vi "Begin.vi"(8 "error in":errorcluster) -> (0 "error out":errorcluster)   [LabVIEW 2015]
doc: "Called before other user functions, this VI is expected to open initial I/O refnums, load in file data, and do all program initialization. Notice that the <B>error out</B> terminal is simply used for data flow. Wiring it to other structures or subVIs ensures that this VI runs first."
uses:
  <vilib>/Rock Robotics/WPI/DriverStation/WPI_DriverStationRobotMode2.ctl
  <vilib>/Rock Robotics/WPI/Joystick/WPI_JoystickDeviceEnum.ctl
  <vilib>/Rock Robotics/WPI/CAN/TalonSRX/WPI_CANTalonSRX_APIControlMode.ctl
  <vilib>/Rock Robotics/WPI/CAN/TalonSRX/WPI_CANTalonSRX_APIFeedbackSelect.ctl
  <vilib>/Rock Robotics/SystemInterfaces/DIO/FPGA_DIOPWMChannel.ctl
  <vilib>/Rock Robotics/WPI/SafetyOutput/WPI_SafetyOutputConfigMenu.ctl
  <vilib>/Rock Robotics/SystemInterfaces/spilib/spi_bus.ctl
  Robot Global Data.vi
  <vilib>/Rock Robotics/WPI/MotorControl/WPI_MotorControlOpenCANTalonSRX.vi
  <vilib>/Rock Robotics/WPI/MotorControl/WPI_MotorControlOpen VictorSP.vi
  <vilib>/Rock Robotics/WPI/Solenoid/WPI_SolenoidOpenSingle.vi
  <vilib>/Rock Robotics/WPI/RobotDrive/WPI_RobotDriveOpen2MotorWithVictorSP.vi
  Z navX/navX Library v2/IO/Open/Z900_navX_Open_SPI.vi
  <vilib>/Rock Robotics/Network Tables/NT Write String Array.vi
  <vilib>/Rock Robotics/WPI/Counter/WPI_CounterDigitalInputToDigitalSource.vi
  <vilib>/Rock Robotics/SystemInterfaces/DIO/FPGA_DIOChannel.ctl
  <vilib>/Rock Robotics/WPI/Encoder/WPI_EncoderType.ctl
  Z navX/navX Library v2/navX Library v2.lvlib
panel:
  in  "I 4":dbl
  in  "F 4":dbl=0.01
  in  "D 4":dbl caption="D"
  in  "P 4":dbl=1.0 caption="P"
  in  "Reverse Feedback Sensor 4":bool
  in  "I 3":dbl
  in  "F 3":dbl=0.01
  in  "D 3":dbl caption="D"
  in  "P 3":dbl=1.0 caption="P"
  in  "Reverse Feedback Sensor 3":bool
  in  "Encoder Codes Per Rev 3":u16=360
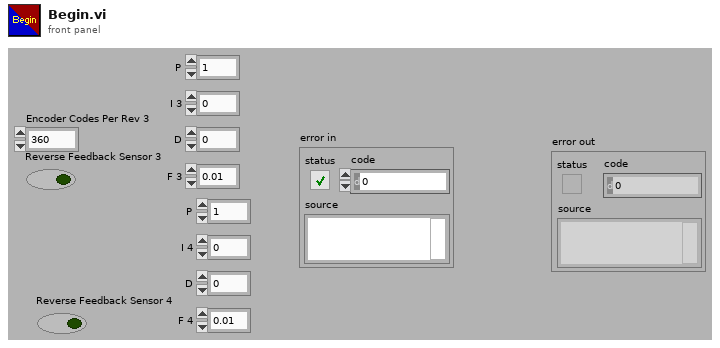
[diagram p1: front panel]
types:
  T1 = typedef "spi_bus.ctl" = enum16{"SPI On-Board, CS0", "SPI On-Board, CS1", "SPI On-Board, CS2", "SPI On-Board, CS3", "SPI MXP", "Invalid"}
  T2 = typedef "WPI_SafetyOutputConfigMenu.ctl" = enum16{"Enable", "Disable"}
  T3 = typedef "FPGA_DIOPWMChannel.ctl" = enum8{"PWM 0", "PWM 1", "PWM 2", "PWM 3", "PWM 4", "PWM 5", "PWM 6", "PWM 7", "PWM 8", "PWM 9", "PWM MXP 0", "PWM MXP 1", "PWM MXP 2", "PWM MXP 3", "PWM MXP 4", "PWM MXP 5", "PWM MXP 6", "PWM MXP 7", "PWM MXP 8", "PWM MXP 9", "Invalid"}
  T4 = typedef "WPI_CANTalonSRX_APIControlMode.ctl" = enum8{"Percent VBus", "Speed", "Position", "Slave", "Unchanged / Invalid", "Voltage Compensation", "Current", "Motion Profile"}
  T5 = typedef "WPI_CANTalonSRX_APIFeedbackSelect.ctl" = enum16{"Digital Quadrature Encoder", "Analog Potentiometer", "Analog Encoder", "Count on Quad-A (Rising-Edge)", "Count on Quad-A (Falling-Edge)", "CTR Magnetic Enc (Absolute)", "CTR Magnetic Enc (Relative)", "Pulse Width"}
  T6 = typedef "WPI_JoystickDeviceEnum.ctl" = enum16{"USB 0", "USB 1", "USB 2", "USB 3", "USB 4", "USB 5"}
  T7 = typedef "WPI_DriverStationRobotMode2.ctl" = enum16{"Autonomous Disabled", "Autonomous Enabled", "Teleop Disabled", "Teleop Enabled", "Disconnected", "Finish", "Test Disabled", "Test Enabled", "Emergency Stopped"}
  T8 = typedef "WPI_SolenoidDevRef.ctl" = cluster{"DevStatus":errorcluster, "Pneumatics Control Module":u8, "Forward Solenoid Channel":T9, "Reverse Solenoid Channel":T9}
  T9 = typedef "WPI_SolenoidChannel.ctl" = enum8{"Solenoid 0", "Solenoid 1", "Solenoid 2", "Solenoid 3", "Solenoid 4", "Solenoid 5", "Solenoid 6", "Solenoid 7", "Invalid"}
  T10 = typedef "WPI_RobotDriveDevRef.ctl" = cluster{"DevStatus":errorcluster, "Motors[]":T11[], "Square Inputs":bool, "Max Output":dbl}
  T11 = typedef "WPI_MotorControlDeviceRef.ctl" = cluster{"DeviceStatus":errorcluster, "Type":T12, "PWM":cluster{"PWM Channel":T3, "DeadBand":T13}, "CAN":cluster{"Device Number":u8, "Control Mode":T14, "Semaphore":T15, "Max Vout":dbl, "TalonSRX Control Mode":T4}, "Invert":bool}
  T12 = typedef "WPI_MotorControlType.ctl" = enum16{"PWM", "CAN", "CANTalonSRX"}
  T13 = typedef "WPI_PWMDeadband.ctl" = cluster{"Name":string, "maxPositivePwm":i32, "minPositivePwm":i32, "centerPwm":i32, "maxNegativePwm":i32, "minNegativePwm":i32, "angularRange":u16}
  T14 = typedef "WPI_CANJaguar_ControlMode.ctl" = enum8{"Percent VBus", "Current", "Speed", "Position", "Voltage"}
  T15 = typedef "Semaphore RefNum" = refnum<k1>
  T16 = typedef "WPI_JoystickDevRef.ctl" = cluster{"Device":T6}
  T17 = typedef "WPI_EncoderType.ctl" = enum16{"1x", "2x", "4x"}
  T18 = typedef "FPGA_DIOChannel.ctl" = enum8{"DIO 0", "DIO 1", "DIO 2", "DIO 3", "DIO 4", "DIO 5", "DIO 6", "DIO 7", "DIO 8", "DIO 9", "DIO MXP 0", "DIO MXP 1", "DIO MXP 2", "DIO MXP 3", "DIO MXP 4", "DIO MXP 5", "DIO MXP 6", "DIO MXP 7", "DIO MXP 8", "DIO MXP 9", "DIO MXP 10", "DIO MXP 11", "DIO MXP 12", "DIO MXP 13", "DIO MXP 14", "DIO MXP 15", "Invalid"}
  T19 = typedef "WPI_DigitalInputDevRef.ctl" = cluster{"DevStatus":errorcluster, "DIO Channel":T18}
  T20 = typedef "FPGA_CounterEncoderSourceConvertionLVSourceType.ctl" = cluster{"DevStatus":errorcluster, "AnalogTriggerMode?":bool, "DigitalMode":cluster{"DIO Channel":T21}, "AnalogTriggerMode":cluster{"AnalogTriggerIndex":T22, "OutputType":T23}}
  T21 = typedef "FPGA_DIODigitalSourceChannel.ctl" = enum8{"DIO 0", "DIO 1", "DIO 2", "DIO 3", "DIO 4", "DIO 5", "DIO 6", "DIO 7", "DIO 8", "DIO 9", "DIO MXP 0", "DIO MXP 1", "DIO MXP 2", "DIO MXP 3", "DIO MXP 4", "DIO MXP 5", "DIO MXP 6", "DIO MXP 7", "DIO MXP 8", "DIO MXP 9", "DIO MXP 10", "DIO MXP 11", "DIO MXP 12", "DIO MXP 13", "DIO MXP 14", "DIO MXP 15", "Disabled"}
  T22 = typedef "FPGA_AnalogTriggerIndex.ctl" = enum8{"Trig 0", "Trig 1", "Trig 2", "Trig 3", "Trig 4", "Trig 5", "Trig 6", "Trig 7", "Invalid"}
  T23 = typedef "FPGA_AnalogTriggerOutType.ctl" = enum16{"InWindow", "TriggerState", "Rising", "Falling"}
  T24 = typedef "WPI_EncoderDevRef.ctl" = cluster{"DevStatus":errorcluster, "EncoderIndex":T25, "CounterIndex":T26, "DistancePerCount":dbl, "Decoding Type":T17}
  T25 = typedef "FPGA_EncoderIdx.ctl" = enum8{"Enc 0", "Enc 1", "Enc 2", "Enc 3", "Enc 4", "Enc 5", "Enc 6", "Enc 7", "Invalid"}
  T26 = typedef "FPGA_CounterCtrSystemIndex.ctl" = enum8{"Ctr 0", "Ctr 1", "Ctr 2", "Ctr 3", "Ctr 4", "Ctr 5", "Ctr 6", "Ctr 7", "Invalid"}
  T27 = typedef "navX Library v2.lvlib/Z900_navX_DeviceTypeDef.ctl" = cluster{"Interface":cluster{"Protocol":T28, "Update Rate (4Hz-60Hz)":u8, "navX Open TypeDef":variant}, "Notify Packet":refnum<notifier>, "Loop VI Refnum":refnum<vi>, "Ready to Close Occurrence Refnum":refnum<k4>}
  T28 = typedef "navX Library v2.lvlib/Z900_navX_ProtocolTypeDef.ctl" = enum16{"SERIAL", "I2C", "SPI"}
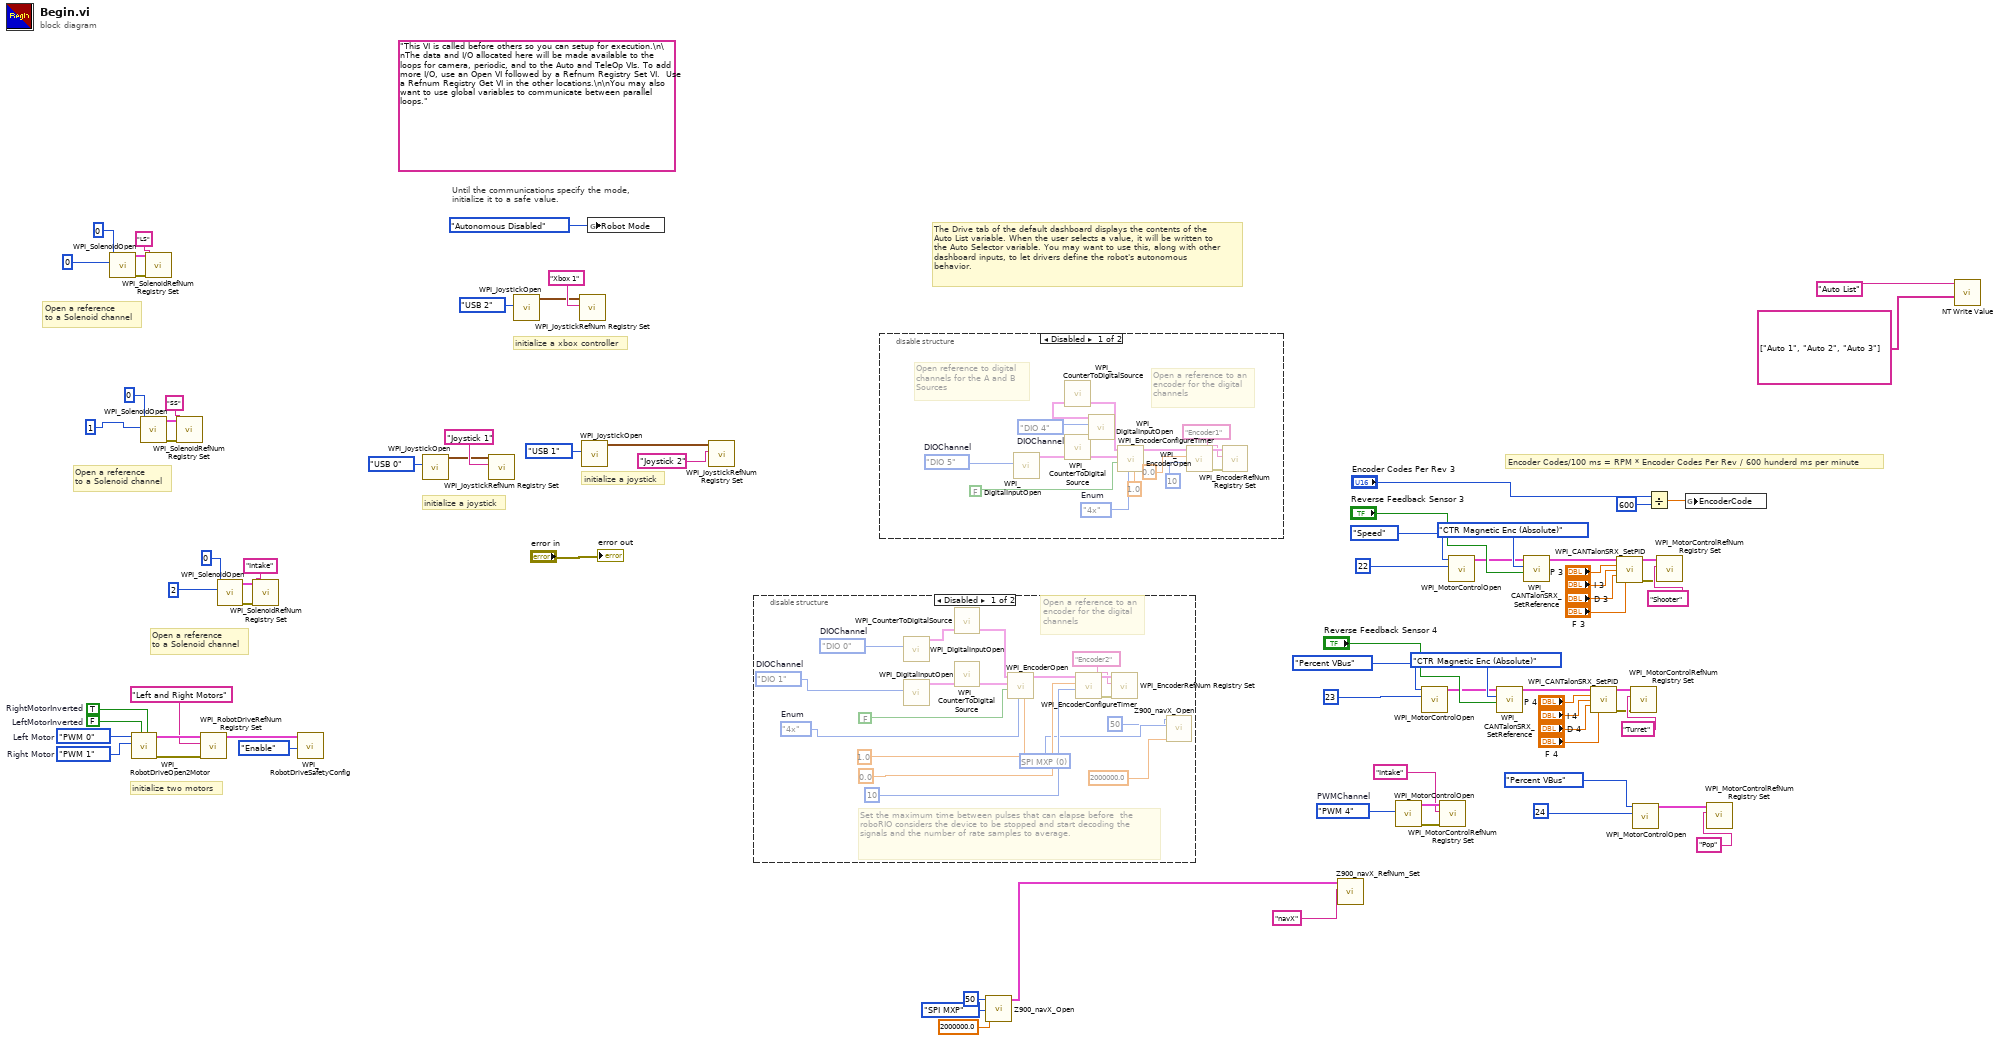
[diagram p0: block diagram]
diagram:
  w10 = FPGA_DIOPWMChannel."PWM 1"  # Right Motor
  w11 = FPGA_DIOPWMChannel."PWM 0"  # Left Motor
  w15 = FALSE  # LeftMotorInverted
  w16 = TRUE  # RightMotorInverted
  w34 = FPGA_DIOPWMChannel."PWM 4"  # PWMChannel
  (unwired) "This VI is called before others so you can setup for execution.\n\nThe data and I/O allocated here will be made available to the loops for camera, periodic, and to the Auto and TeleOp VIs. To add more I/O, use an Open VI followed by a Refnum Registry Set VI.  Use a Refnum Registry Get VI in the other locations.\n\nYou may also want to use global variables to communicate between parallel loops."
  # "initialize two motors"
  # "Open a reference \nto a Solenoid channel"
  # "Open a reference \nto a Solenoid channel"
  # "Open a reference \nto a Solenoid channel"
  # "Encoder Codes/100 ms = RPM * Encoder Codes Per Rev / 600 hunderd ms per minute"
  # "initialize a xbox controller"
  # "The Drive tab of the default dashboard displays the contents of the\nAuto List variable. When the user selects a value, it will be written to\nthe Auto Selector variable. You may want to use this, along with other\ndashboard inputs, to let drivers define the robot's autonomous\nbehavior."
  # "initialize a joystick"
  # "initialize a joystick"
  # "Until the communications specify the mode,\ninitialize it to a safe value."
  n1 = call-poly <vilib>:"WPI_SolenoidOpen.vi"("Solenoid Channel"=0, "Pneumatics Control Module (0)"=0) -> ("error out"=w23:errorcluster, "SolenoidDevRef"=w22:T8)  [unwired: 1 in, 7 out]
  n2 = call-poly <vilib>:"WPI_RobotDriveOpen2Motor.vi"("Right Motor Inverted"=w16, "Left Motor Inverted"=w15, "Right Motor"=w10, "Left Motor"=w11) -> ("error out"=w12:errorcluster, "RobotDriveDevRef"=w14:T10)  [unwired: 1 in, 5 out]
  n3 = call-poly <vilib>:"WPI_SolenoidOpen.vi"("Solenoid Channel"=1, "Pneumatics Control Module (0)"=0) -> ("error out"=w27:errorcluster, "SolenoidDevRef"=w26:T8)  [unwired: 1 in, 7 out]
  n4 = call <vilib>:"WPI_SolenoidRefNum Registry Set.vi"("error in (no error)"=w23, "refnum name"="LS", "SolenoidDevRef"=w22) -> ()  [unwired: 7 in, 2 out]
  n5 = call <vilib>:"WPI_SolenoidRefNum Registry Set.vi"("error in (no error)"=w27, "refnum name"="SS", "SolenoidDevRef"=w26) -> ()  [unwired: 7 in, 2 out]
  n6 = call <vilib>:"WPI_RobotDriveRefNum Registry Set.vi"("error in (no error)"=w12, "refnum name"="Left and Right Motors", "RobotDriveDevRef"=w14) -> ("RobotDriveDevRef"=w9:T10)  [unwired: 1 in, 7 out]
  n7 = call-poly <vilib>:"WPI_SolenoidOpen.vi"("Solenoid Channel"=2, "Pneumatics Control Module (0)"=0) -> ("error out"=w31:errorcluster, "SolenoidDevRef"=w30:T8)  [unwired: 1 in, 7 out]
  n8 = call <vilib>:"WPI_SolenoidRefNum Registry Set.vi"("error in (no error)"=w31, "refnum name"="Intake", "SolenoidDevRef"=w30) -> ()  [unwired: 7 in, 2 out]
  n9 = call <vilib>:"WPI_RobotDriveSafetyConfig.vi"("mode"=WPI_SafetyOutputConfigMenu."Enable", "RobotDriveDevRef"=w9) -> ()  [unwired: 8 in, 2 out]
  n10 = call <vilib>:"WPI_JoystickOpen.vi"("JoystickDevice"=WPI_JoystickDeviceEnum."USB 0") -> ("JoystickDevRef"=w76:T16)  [unwired: 10 in]
  n11 = call <vilib>:"WPI_JoystickRefNum Registry Set.vi"("refnum name"="Joystick 1", "JoystickDevRef"=w76) -> ()  [unwired: 8 in, 2 out]
  n12 = call <vilib>:"WPI_JoystickOpen.vi"("JoystickDevice"=WPI_JoystickDeviceEnum."USB 2") -> ("JoystickDevRef"=w70:T16)  [unwired: 10 in]
  n13 = call <vilib>:"WPI_JoystickRefNum Registry Set.vi"("refnum name"="Xbox 1", "JoystickDevRef"=w70) -> ()  [unwired: 8 in, 2 out]
  n14 = call <vilib>:"WPI_JoystickOpen.vi"("JoystickDevice"=WPI_JoystickDeviceEnum."USB 1") -> ("JoystickDevRef"=w73:T16)  [unwired: 10 in]
  n15 = global write "Robot Global Data.vi" "Robot Mode"(WPI_DriverStationRobotMode2."Autonomous Disabled" ("Robot Mode")) -> ()
  n16 = call <vilib>:"WPI_JoystickRefNum Registry Set.vi"("refnum name"="Joystick 2", "JoystickDevRef"=w73) -> ()  [unwired: 8 in, 2 out]
  n17 = disable-structure shown="Disabled" {
    frame Disabled {
      w82 = u16 0 items=["SPI MXP", "SPI On-Board, CS0"]
      w86 = WPI_EncoderType."4x"  # Enum
      w88 = FPGA_DIOChannel."DIO 1"  # DIOChannel
      w89 = FPGA_DIOChannel."DIO 0"  # DIOChannel
      # "Set the maximum time between pulses that can elapse before  the roboRIO considers the device to be stopped and start decoding the signals and the number of rate samples to average."
      # "Open a reference to an\nencoder for the digital \nchannels"
      n18 = call <vilib>:"WPI_DigitalInputOpen.vi"("DIO Channel"=w89) -> ("DigitalInputDevRef"=w95:T19)  [unwired: 1 in, 9 out]
      n19 = call <vilib>:"WPI_DigitalInputOpen.vi"("DIO Channel"=w88) -> ("DigitalInputDevRef"=w96:T19)  [unwired: 1 in, 9 out]
      n20 = call-poly <vilib>:"WPI_CounterToDigitalSource.vi"("DigitalInputDevRef"=w95) -> ("Digital Source"=w94:T20)  [unwired: 6 out]
      n21 = call-poly <vilib>:"WPI_CounterToDigitalSource.vi"("DigitalInputDevRef"=w96) -> ("Digital Source"=w97:T20)  [unwired: 6 out]
      n22 = call <vilib>:"WPI_EncoderOpen.vi"("DistancePerCount"=1.0, "Decoding Type"=w86, "Invert Direction (False)"=FALSE, "BSource"=w97, "ASource"=w94) -> ("EncoderDevRef"=w93:T24)  [unwired: 3 in, 3 out]
      n23 = call <vilib>:"WPI_EncoderConfigureTimer.vi"("Number Samples to Average"=10, "Minimum Rate"=0.0, "EncoderDevRef"=w93) -> ("error out"=w92:errorcluster, "EncoderDevRef"=w91:T24)  [unwired: 1 in, 6 out]
      n24 = call <vilib>:"WPI_EncoderRefNum Registry Set.vi"("error in (no error)"=w92, "refnum name"="Encoder2", "EncoderDevRef"=w91) -> ()  [unwired: 7 in, 2 out]
      n25 = call-poly "Z900_navX_Open.vi"("Clock Rate (Hz)"=2000000.0, "SPI Bus"=w82, "Update Rate (4Hz-60Hz)"=50) -> ()  [unwired: 7 in, 2 out]
    }
    frame Enabled {
    }
  }
  n26 = disable-structure shown="Disabled" {
    frame Disabled {
      w101 = WPI_EncoderType."4x"  # Enum
      w103 = FPGA_DIOChannel."DIO 5"  # DIOChannel
      w104 = FPGA_DIOChannel."DIO 4"  # DIOChannel
      # "Open a reference to an\nencoder for the digital \nchannels"
      # "Open reference to digital \nchannels for the A and B\nSources"
      n27 = call <vilib>:"WPI_DigitalInputOpen.vi"("DIO Channel"=w103) -> ("DigitalInputDevRef"=w111:T19)  [unwired: 1 in, 9 out]
      n28 = call-poly <vilib>:"WPI_CounterToDigitalSource.vi"("DigitalInputDevRef"=w111) -> ("Digital Source"=w112:T20)  [unwired: 6 out]
      n29 = call <vilib>:"WPI_DigitalInputOpen.vi"("DIO Channel"=w104) -> ("DigitalInputDevRef"=w110:T19)  [unwired: 1 in, 9 out]
      n30 = call-poly <vilib>:"WPI_CounterToDigitalSource.vi"("DigitalInputDevRef"=w110) -> ("Digital Source"=w109:T20)  [unwired: 6 out]
      n31 = call <vilib>:"WPI_EncoderOpen.vi"("DistancePerCount"=1.0, "Decoding Type"=w101, "Invert Direction (False)"=FALSE, "BSource"=w112, "ASource"=w109) -> ("EncoderDevRef"=w108:T24)  [unwired: 3 in, 3 out]
      n32 = call <vilib>:"WPI_EncoderConfigureTimer.vi"("Number Samples to Average"=10, "Minimum Rate"=0.0, "EncoderDevRef"=w108) -> ("error out"=w107:errorcluster, "EncoderDevRef"=w106:T24)  [unwired: 1 in, 6 out]
      n33 = call <vilib>:"WPI_EncoderRefNum Registry Set.vi"("error in (no error)"=w107, "refnum name"="Encoder1", "EncoderDevRef"=w106) -> ()  [unwired: 7 in, 2 out]
    }
    frame Enabled {
    }
  }
  n34 = call-poly "Z900_navX_Open.vi"("Clock Rate (Hz)"=2000000.0, "SPI Bus"=spi_bus."SPI MXP", "Update Rate (4Hz-60Hz)"=u8 50) -> ("navX Device"=w3:T27)  [unwired: 7 in, 1 out]
  n35 = call "Z900_navX_RefNum_Set.vi"("refnum name"="navX", "navX Device"=w3) -> ()  [unwired: 8 in, 2 out]
  n36 = call-poly <vilib>:"WPI_MotorControlOpen.vi"("PWM Channel"=w34) -> ("error out"=w36:errorcluster, "MotorControlDeviceRef"=w35:T11)  [unwired: 9 in]
  n37 = call-poly <vilib>:"WPI_MotorControlOpen.vi"("Device Number"=23, "Control Mode"=WPI_CANTalonSRX_APIControlMode."Percent VBus") -> ("MotorControlDeviceRef"=w48:T11)  [unwired: 3 in, 6 out]
  n38 = call <vilib>:"WPI_MotorControlRefNum Registry Set.vi"("error in (no error)"=w36, "refnum name"="Intake", "MotorControlDevRef"=w35) -> ()  [unwired: 7 in, 2 out]
  n39 = call-poly <vilib>:"WPI_MotorControlOpen.vi"("Device Number"=22, "Control Mode"=WPI_CANTalonSRX_APIControlMode."Speed") -> ("MotorControlDeviceRef"=w61:T11)  [unwired: 3 in, 6 out]
  n40 = call <vilib>:"WPI_CANTalonSRX_SetReference.vi"("Reverse Feedback Sensor"="Reverse Feedback Sensor 4", "Feedback Reference"=WPI_CANTalonSRX_APIFeedbackSelect."CTR Magnetic Enc (Absolute)", "CAN Talon SRX Ref"=w48) -> ("CAN Talon SRX Ref"=w47:T11)  [unwired: 7 in, 1 out]
  n41 = call <vilib>:"WPI_CANTalonSRX_SetReference.vi"("Reverse Feedback Sensor"="Reverse Feedback Sensor 3", "Feedback Reference"=WPI_CANTalonSRX_APIFeedbackSelect."CTR Magnetic Enc (Absolute)", "CAN Talon SRX Ref"=w61) -> ("CAN Talon SRX Ref"=w60:T11)  [unwired: 7 in, 1 out]
  n42 = call <vilib>:"WPI_CANTalonSRX_SetPID.vi"("CAN Talon SRX Ref"=w47, "P"="P 4", "I"="I 4", "D"="D 4", "F"="F 4") -> ("CAN Talon SRX Ref"=w44:T11, "error out"=w42:errorcluster)  [unwired: 9 in]
  n43 = call <vilib>:"WPI_CANTalonSRX_SetPID.vi"("CAN Talon SRX Ref"=w60, "P"="P 3", "I"="I 3", "D"="D 3", "F"="F 3") -> ("CAN Talon SRX Ref"=w56:T11, "error out"=w54:errorcluster)  [unwired: 9 in]
  n44 = call <vilib>:"WPI_MotorControlRefNum Registry Set.vi"("error in (no error)"=w42, "refnum name"="Turret", "MotorControlDevRef"=w44) -> ()  [unwired: 7 in, 2 out]
  n45 = call-poly <vilib>:"WPI_MotorControlOpen.vi"("Device Number"=24, "Control Mode"=WPI_CANTalonSRX_APIControlMode."Percent VBus") -> ("MotorControlDeviceRef"=w32:T11)  [unwired: 3 in, 6 out]
  n46 = Divide(x="Encoder Codes Per Rev 3", y=u16 600) -> (x/y=w57:dbl)
  n47 = call <vilib>:"WPI_MotorControlRefNum Registry Set.vi"("error in (no error)"=w54, "refnum name"="Shooter", "MotorControlDevRef"=w56) -> ()  [unwired: 7 in, 2 out]
  n48 = global write "Robot Global Data.vi" "EncoderCode"(w57) -> ()
  n49 = call <vilib>:"WPI_MotorControlRefNum Registry Set.vi"("refnum name"="Pop", "MotorControlDevRef"=w32) -> ()  [unwired: 8 in, 2 out]
  n50 = call-poly <vilib>:"NT Write Value.vi"("String Array"=string[] ["Auto 1", "Auto 2", "Auto 3"], "Name"="Auto List") -> ()  [unwired: 9 in, 1 out]
  "error out" <- "error in"
